vi "Get Object Name.vi"(8 "error in (no error)":errorcluster, 11 "Storage Object in":refnum<k20>) -> (0 "error out":errorcluster, 2 "Name":string, 3 "Storage Object out":refnum<k20>)   [LabVIEW 2015, in "Engine Simulation Toolkit System Explorer.lvlib" / "File Interface.lvlib"]
uses:
  File Interface.lvlib
  <vilib>/Platform/storage/Storage.llb/Get Property (String).vi
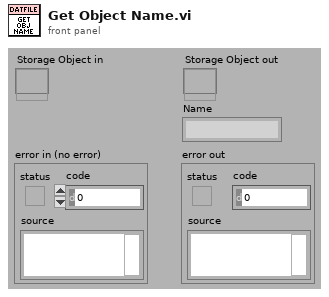
[diagram p1: front panel]
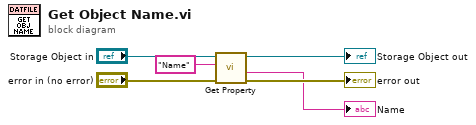
[diagram p0: block diagram]
diagram:
  n1 = call-poly <vilib>:"Get Property.vi"("error in (no error)"="error in (no error)", "Property name"="Name" ("PropertyName"), "storage refnum"="Storage Object in") -> ("error out"=→"error out":errorcluster, "Value"=→"Name":string, "storage refnum out"=→"Storage Object out":refnum<k20>)  [unwired: 6 out]
